vi "Verify Unique Device.vi"(8 "error in (no error)":errorcluster, 10 "Device":string, 11 "Configuration in":refnum<class "Configuration.lvclass">) -> (0 "error out":errorcluster, 2 "Name Added":bool, 3 "Configuration out":refnum<class "Configuration.lvclass">)   [LabVIEW 2023, in "Configuration.lvlib" / "Configuration.lvclass"]
uses:
  Library/Configuration.lvclass
  Library/Configuration.lvclass/Configuration.ctl
  <vilib>/Utility/error.llb/Trim Whitespace One-Sided.vi
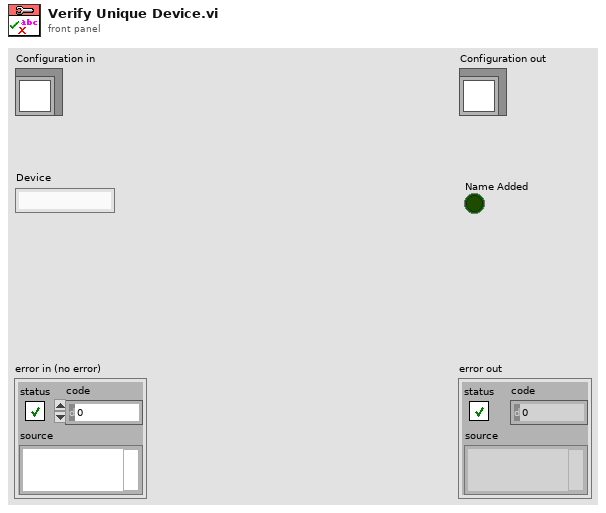
[diagram p1: front panel]
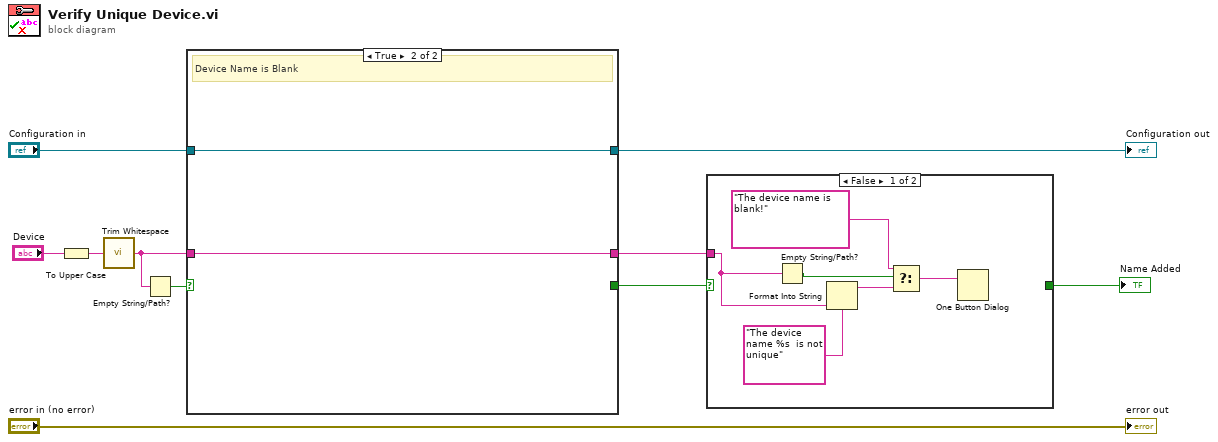
[diagram p0: block diagram]
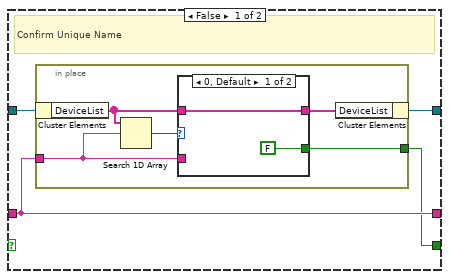
[diagram p3: hidden frame]
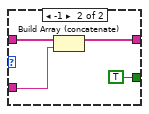
[diagram p4: hidden frame]
diagram:
  n1 = To Upper Case(1:"Device") -> (0:w9:string)
  n2 = call <vilib>:"Trim Whitespace.vi"("string"=w9) -> ("trimmed string"=w6:string)  [unwired: 1 in]
  n3 = Empty String/Path?(string/path=w6) -> (empty?=w7:bool)
  n4 = case shown="True" w7 {
    tunnel: w6 -> [w12 w26]
    tunnel: [w11 _] -> w5
    tunnel: "Configuration in" -> [w14 w27]
    tunnel: [w13 w27] -> w3
    tunnel: [w12 w26] -> w1
    frame False {
      # "Confirm Unique Name"
      n5 = in-place {
        in-place-border: w12 -> [w15]
        in-place-border: [w16] -> w11
        n6 = in-place-cluster #1(w14) -> ("DeviceList"=w18:string[])
        n7 = Search 1D Array(1D array=w18, element=w15) -> (index of element=w19:i32)  [unwired: 1 in]
        n8 = case shown="0, Default" w19 {
          tunnel: w18 -> [w21 w25]
          tunnel: [w21 w24] -> w17
          tunnel: [FALSE TRUE] -> w16
          tunnel: w15 -> [_ w23]
          frame 0, Default {
          }
          frame -1 {
            n9 = Build Array (concatenate)(w25, w23) -> (w24:string[])
          }
        }
        n10 = in-place-cluster #1("DeviceList"=w17) -> (w13:refnum<class "Configuration.lvclass">)
      }
    }
    frame True {
      # "Device Name is Blank"
    }
  }
  "Configuration out" <- w3
  n11 = case shown="False" w5 {
    selector: w5 -> [_ w34]
    tunnel: [_ w34] -> w2
    tunnel: w1 -> [w30 _]
    frame False {
      n12 = Empty String/Path?(string/path=w30) -> (empty?=w31:bool)
      n13 = Format Into String(format string="The device name %s  is not unique", w30) -> (resulting string=w29:string)  [unwired: 2 in, 1 out]
      n14 = Select(t="The device name is blank!", s=w31, f=w29) -> (s? t:f=w32:string)
      n15 = One Button Dialog(message=w32) -> ()  [unwired: 1 in, 1 out]
    }
    frame True {
    }
  }
  "Name Added" <- w2
  "error out" <- "error in (no error)"
